vi "Set Properties.vi"(8 "error in (no error)":errorcluster, 10 "Properties":T1[](array[typedef]), 11 "CycloneDX JSON in":refnum<class "CycloneDX JSON.lvclass">) -> (0 "error out":errorcluster, 3 "CycloneDX JSON out":refnum<class "CycloneDX JSON.lvclass">)   [LabVIEW 2017, in "LabVIEW CycloneDX SBOM.lvlib" / "CycloneDX JSON.lvclass"]
doc: "Sets properties (name-value pairs) as $.properties path of the JSON representation."
uses:
  CycloneDX JSON.lvclass
  Name Value Pair.ctl
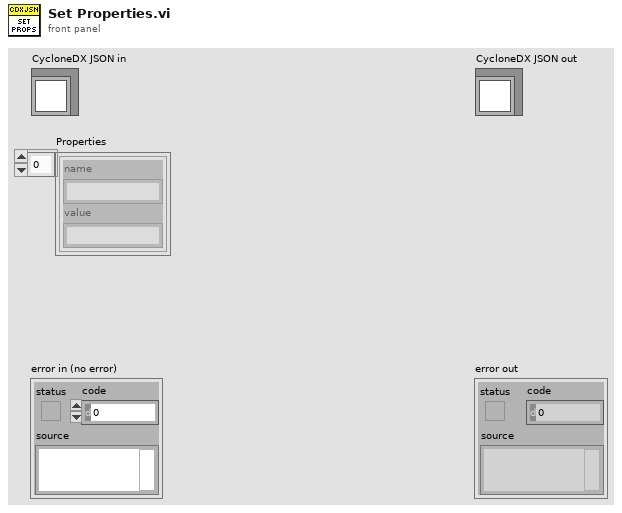
[diagram p1: front panel]
types:
  T1 = typedef "LabVIEW CycloneDX SBOM.lvlib/CycloneDX JSON.lvclass/Name Value Pair.ctl" = cluster{"name":string, "value":string}
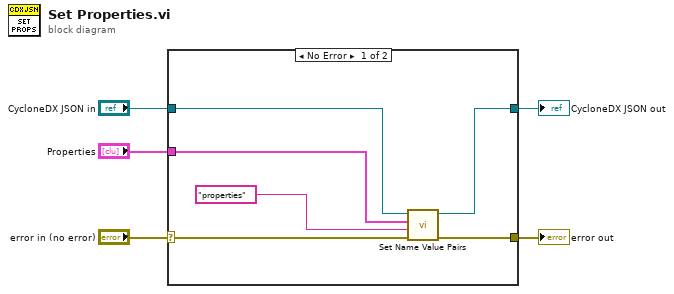
[diagram p0: block diagram]
diagram:
  n1 = case shown="No Error" "error in (no error)" {
    selector: "error in (no error)" -> [w8 w13]
    tunnel: [w7 w13] -> w4
    tunnel: [w9 w12] -> w2
    tunnel: "CycloneDX JSON in" -> [w10 w12]
    tunnel: "Properties" -> [w6 _]
    frame No Error {
      n2 = call "Set Name Value Pairs.vi"("error in (no error)"=w8, "Object (or Item) Path"="properties", "Properties"=w6, "CycloneDX JSON in"=w10) -> ("error out"=w7:errorcluster, "CycloneDX JSON out"=w9:refnum<class "CycloneDX JSON.lvclass">)  [unwired: 6 in]
    }
    frame Error {
    }
  }
  "error out" <- w4
  "CycloneDX JSON out" <- w2
